vi "qc5psmCurrent1.vi"() -> ()   [LabVIEW 2020]
uses:
  <instrlib>/CAEN PSM/CAEN PSM.lvlib
panel:
  in  "Tab Control":enum32{"Page 1"}(tab)
  out "RAMPUP1TIME":dbl
  in  "Tab Control 2":enum32{"Page 1", "Page 2"}(tab)
  out "V monitor":dbl(graph)
  out "I monitor":dbl(graph)
  out "Actual voltage level (Vmon)":dbl
  out "Actual current level (Imon)":dbl
  in  "I_step":dbl=10.0
  in  "VISA resource name":refnum<visa-resource-name>
  in  "Voltage ramp up (0 V/s)":u16 max=999
  in  "Voltage Max (0.0 V)":u16 max=9999
  in  "Board Address":i8 max=31
  out "Vset_initial":dbl=100.0
  out "OVV 2":bool
  out "OVC 2":bool
  out "R calc":dbl
  in  "START AGAIN":bool
  out "Channel Status Array":T1(array[cluster])
  in  "Channel (0)":u8=1
  in  "Req (Mohm)":dbl=4.647
  out "I set status":dbl
  in  "stop":bool
  in  "I_initial":dbl=550.0
  in  "wait for user to next reading":bool
  in  "I _Max":dbl=730.0
  out "status":string
  out "ENTER TIME RAMP VAL":i32
  out "RDW":bool
  out "Actual I mon STOP":dbl
  out "In Range?":bool
  out "INNER  RAMP VAL":dbl
  out "CURRENT INCREASE/DECREASE  PER 1 VOLT":dbl
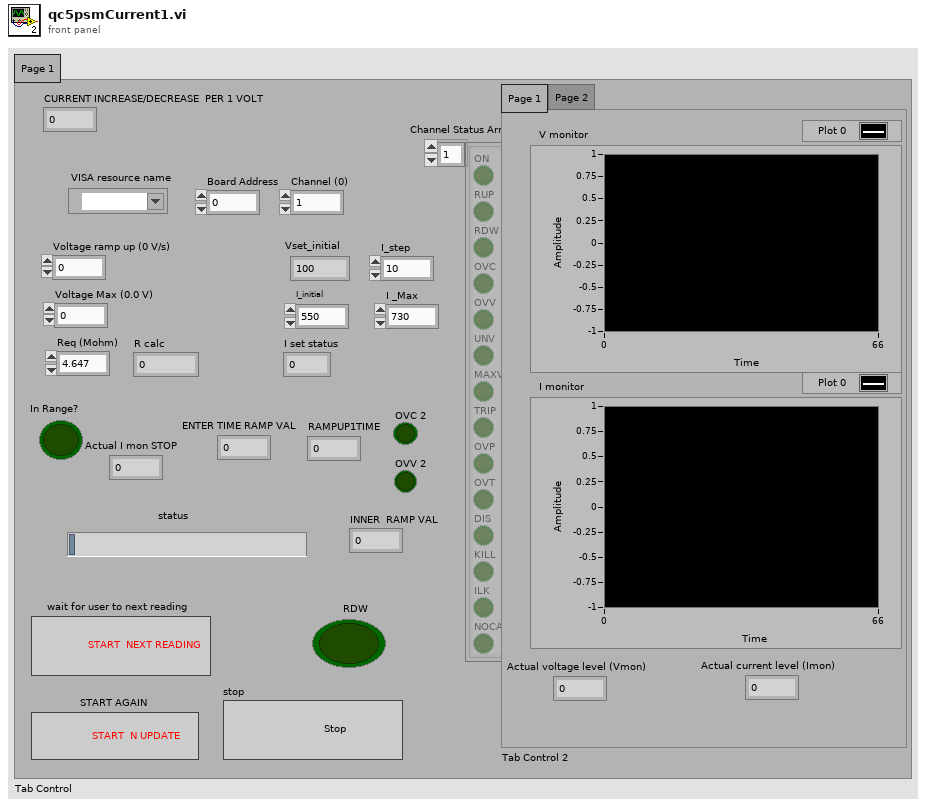
[diagram p1: front panel]
types:
  T1 = cluster{"ON":bool, "RUP":bool, "RDW":bool, "OVC":bool, "OVV":bool, "UNV":bool, "MAXV":bool, "TRIP":bool, "OVP":bool, "OVT":bool, "DIS":bool, "KILL":bool, "ILK":bool, "NOCAL":bool}[]
  T2 = cluster{"Baud Rate":u32, "Parity":enum16{"None", "Odd", "Even", "Mark", "Space"}, "Data Bits":u16, "Stop Bits":u16, "Flow Control":u16}
  T3 = typedef "CAEN PSM.lvlib/BoardHandle.ctl" = cluster{"VISA resource name":refnum<visa-resource-name>, "Board address":i8, "NChannels":u8}
  T4 = cluster{"ON":bool, "RUP":bool, "RDW":bool, "OVC":bool, "OVV":bool, "UNV":bool, "MAXV":bool, "TRIP":bool, "OVP":bool, "OVT":bool, "DIS":bool, "KILL":bool, "ILK":bool, "NOCAL":bool}
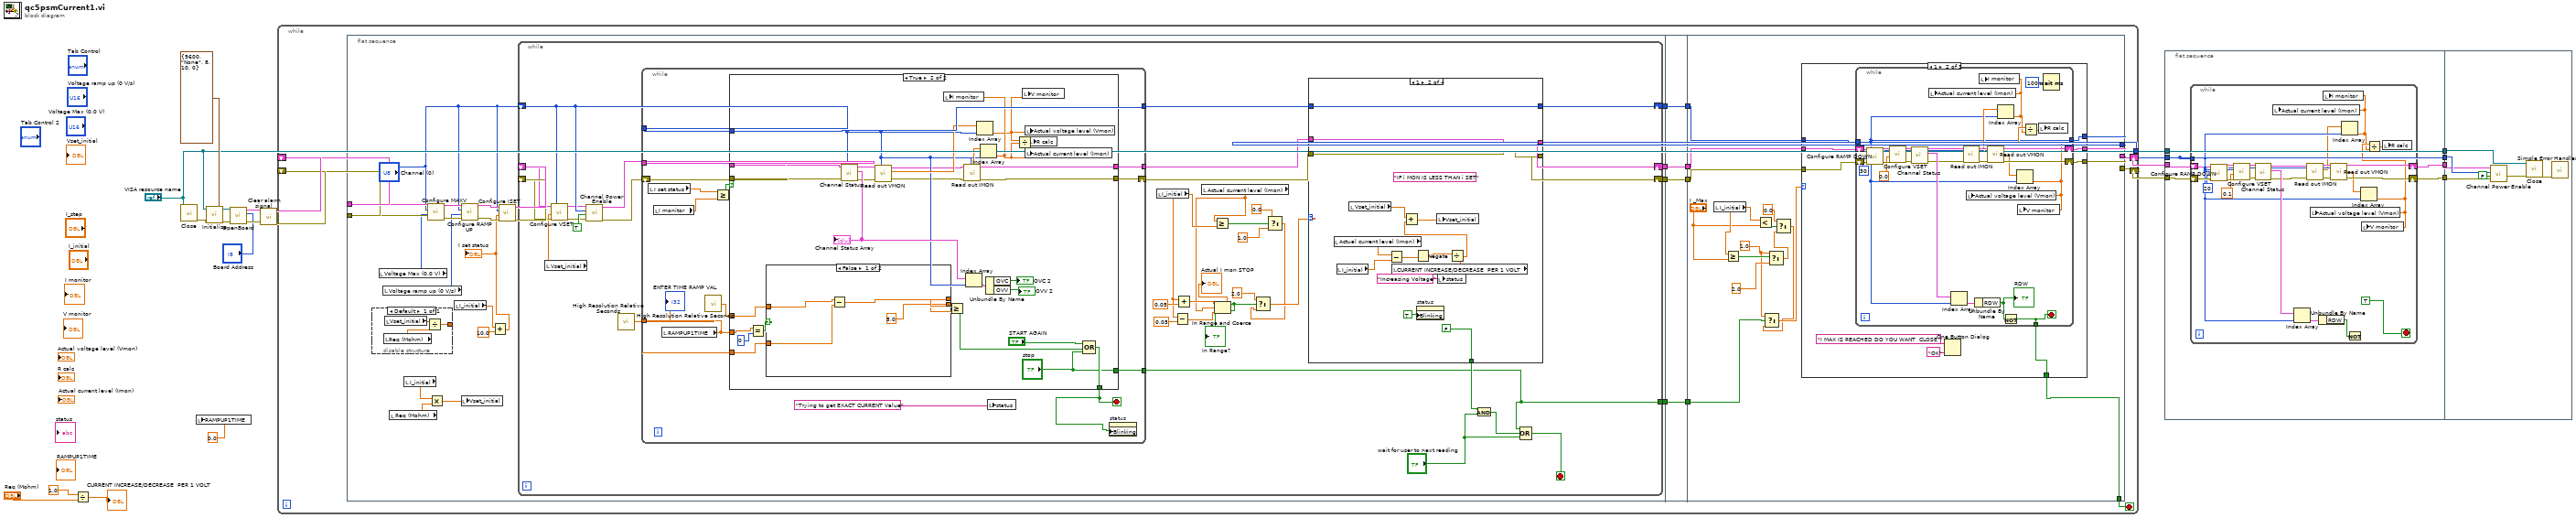
[diagram p0: block diagram]
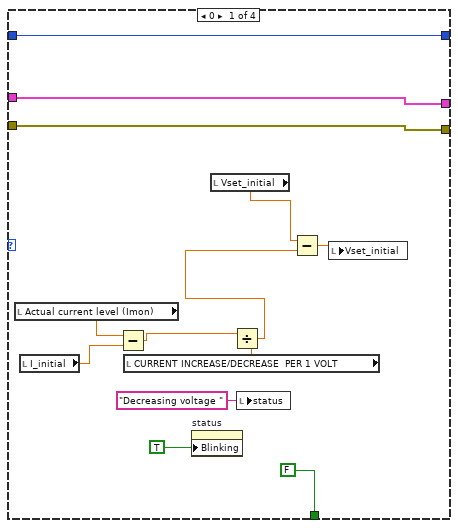
[diagram p2: hidden frame]
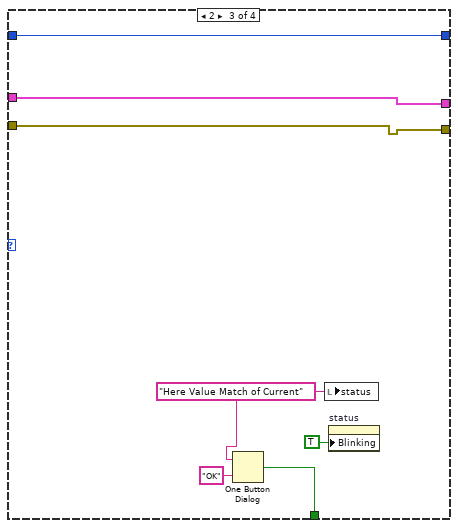
[diagram p3: hidden frame]
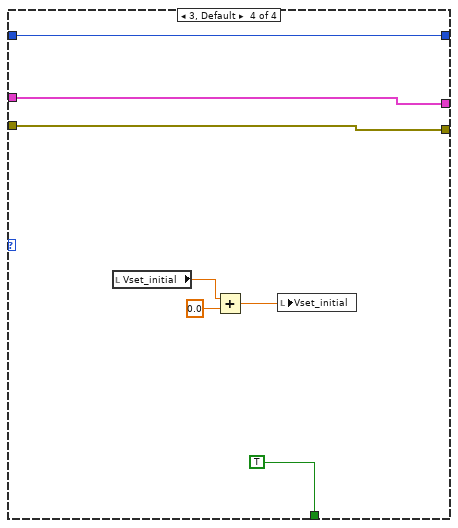
[diagram p4: hidden frame]
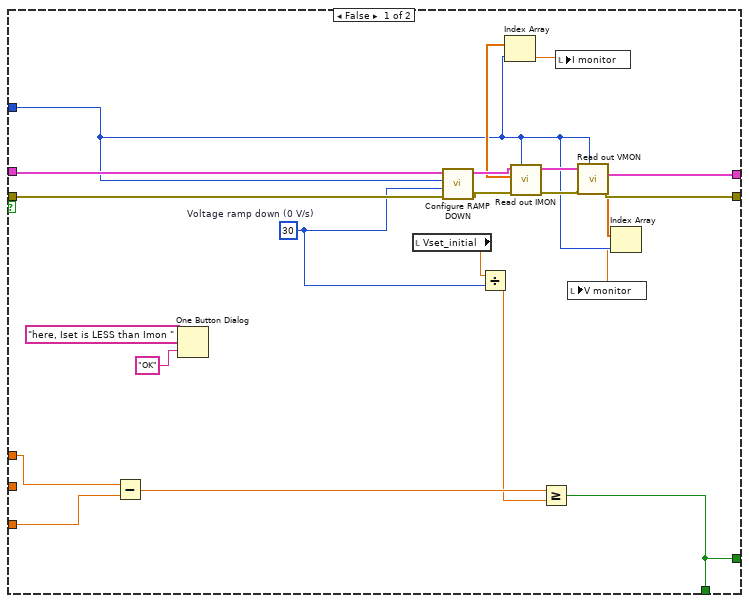
[diagram p5: hidden frame]
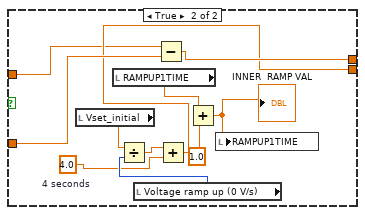
[diagram p6: hidden frame]
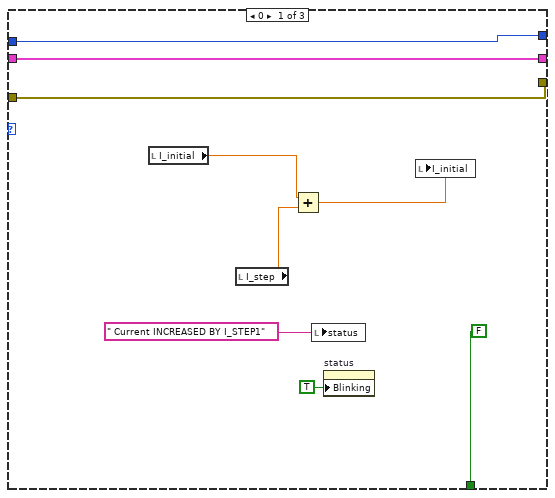
[diagram p7: hidden frame]
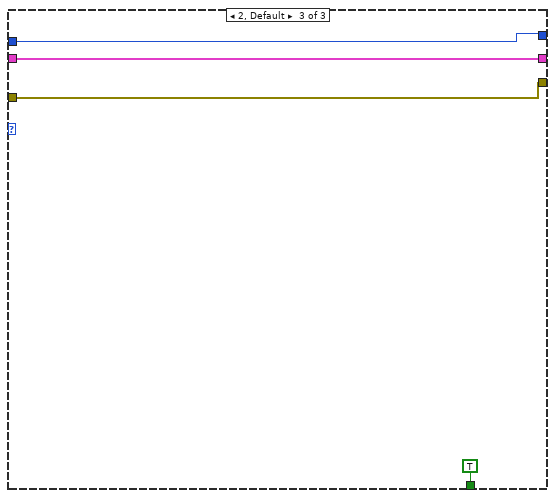
[diagram p8: hidden frame]
diagram:
  n1 = Divide(x=1.0, y="Req (Mohm)") -> (x/y=→"CURRENT INCREASE/DECREASE  PER 1 VOLT":dbl)
  n2 = call <instrlib>:"Close.vi"("VISA resource name"="VISA resource name") -> ("error out"=w12:errorcluster)  [unwired: 10 in]
  n3 = local write "RAMPUP1TIME"(0.0 ("RAMPUP1TIME")) -> ()
  n4 = call <instrlib>:"Initialize.vi"("Serial Configuration"=T2 {"Baud Rate"=9600, "Parity"=enum."None", "Data Bits"=8, "Stop Bits"=10, "Flow Control"=0}, "error in (no error)"=w12, "VISA resource name"="VISA resource name") -> ("error out"=w11:errorcluster, "VISA resource name out"=w20:refnum<visa-resource-name>)  [unwired: 7 in]
  n5 = call <instrlib>:"OpenBoard.vi"("error in (no error)"=w11, "Board Address"="Board Address", "VISA resource name"=w20) -> ("error out"=w18:errorcluster, "BoardHandle"=w19:T3)  [unwired: 7 in]
  n6 = call <instrlib>:"Clear alarm signal.vi"("error in (no error)"=w18, "BoardHandle"=w19) -> ("error out"=w13:errorcluster, "BoardHandle out"=w14:T3)  [unwired: 8 in]
  n7 = while {
    tunnel: [w35] -> w15
    shift-right: [w32] -> w10
    shift-left: w14 -> [w34]
    shift-right: [w30] -> w9
    shift-left: w13 -> [w33]
    stop <- w31 stop-if-true
    n8 = flat-sequence {
      tunnel: w34 -> [w55]
      tunnel: w33 -> [w54]
      tunnel: [w56] -> w25
      tunnel: [w43] -> w27
      tunnel: [w42] -> w29
      tunnel: [w36] -> w23
      tunnel: w29 -> [w219]
      tunnel: [w219] -> w28
      tunnel: w27 -> [w218]
      tunnel: [w218] -> w26
      tunnel: w25 -> [w217]
      tunnel: [w217] -> w24
      tunnel: w23 -> [w216]
      tunnel: [w216] -> w22
      tunnel: [w232] -> w30
      tunnel: [w231] -> w32
      tunnel: [w225] -> w35
      tunnel: [w224] -> w31
      tunnel: w28 -> [w229]
      tunnel: w26 -> [w228]
      tunnel: w24 -> [w230]
      tunnel: w22 -> [w223]
      frame #0 {
        n9 = disable-structure shown="Default" {
          disable-tunnel: [w59] -> _
          frame Enabled {
            n10 = local read "Req (Mohm)"() -> (w57:dbl)
            n11 = local read "Vset_initial"() -> (w58:dbl)
            n12 = Divide(x=w58, y=w57) -> (x/y=w59:dbl)
          }
        }
        n13 = local read "Voltage Max (0.0 V)"() -> (w51:u16)
        n14 = local read "Voltage ramp up (0 V/s)"() -> (w50:u16)
        n15 = local read "Req (Mohm)"() -> (w39:dbl)
        n16 = local read "I_initial"() -> (w38:dbl)
        n17 = call <instrlib>:"Configure MAXV.vi"("error in (no error)"=w54, "Voltage Max (0.0 V)"=w51, "Channel (0)"="Channel (0)", "BoardHandle"=w55) -> ("error out"=w52:errorcluster, "BoardHandle out"=w53:T3)  [unwired: 6 in]
        n18 = Multiply(x=w38, y=w39) -> (x*y=w40:dbl)
        n19 = local read "I_initial"() -> (w37:dbl)
        n20 = local write "Vset_initial"(w40) -> ()
        n21 = call <instrlib>:"Configure RAMP UP.vi"("error in (no error)"=w52, "Voltage ramp up (0 V/s)"=w50, "Channel (0)"="Channel (0)", "BoardHandle"=w53) -> ("error out"=w47:errorcluster, "BoardHandle out"=w49:T3)  [unwired: 6 in]
        n22 = Add(x=w37, y=10.0) -> (x+y=w41:dbl)
        "I set status" <- w41
        n23 = call <instrlib>:"Configure ISET.vi"("error in (no error)"=w47, "Current Limit (0.00 uA)"=w41, "Channel (0)"="Channel (0)", "BoardHandle"=w49) -> ("error out"=w46:errorcluster, "BoardHandle out"=w48:T3)  [unwired: 6 in]
        n24 = while {
          shift-right: [w73] -> w43
          shift-left: w48 -> [w91]
          shift-right: [w71] -> w42
          shift-left: w46 -> [w90]
          shift-right: [w75] -> w56
          shift-left: "Channel (0)" -> [w89]
          tunnel: [w77] -> w36
          stop <- w78 stop-if-true
          n25 = local read "Vset_initial"() -> (w83:dbl)
          n26 = call <instrlib>:"Configure VSET.vi"("error in (no error)"=w90, "Voltage Level (0.0 V)"=w83, "Channel (0)"=w89, "BoardHandle"=w91) -> ("error out"=w88:errorcluster, "BoardHandle out"=w87:T3)  [unwired: 6 in]
          n27 = call <instrlib>:"Channel Power Enable.vi"("error in (no error)"=w88, "Enable (OFF)"=TRUE, "Channel (0)"=w89, "BoardHandle"=w87) -> ("error out"=w93:errorcluster, "BoardHandle out"=w94:T3)  [unwired: 6 in]
          n28 = call <vilib>:"High Resolution Relative Seconds.vi"() -> ("relative seconds"=w86:dbl)
          n29 = while {
            shift-right: [w146] -> w72
            shift-left: w93 -> [w147]
            tunnel: [w145] -> w74
            tunnel: [w149] -> w76
            tunnel: w94 -> [w148]
            tunnel: w89 -> [w149]
            tunnel: w86 -> [w143]
            tunnel: [w139] -> w77
            stop <- w137 stop-if-true
            n30 = local read "I set status"() -> (w142:dbl)
            n31 = local read "I monitor"() -> (w140:dbl)
            n32 = local read "RAMPUP1TIME"() -> (w136:dbl)
            "ENTER TIME RAMP VAL" <- w136
            n33 = call <vilib>:"High Resolution Relative Seconds.vi"() -> ("relative seconds"=w141:dbl)
            n34 = Greater Or Equal?(x=w142, y=w140) -> (x >= y?=w144:bool)
            n35 = case shown="True" w144 {
              tunnel: w149 -> [w156 w194]
              tunnel: w148 -> [w171 w193]
              tunnel: w147 -> [w170 w192]
              tunnel: [w159 w191] -> w146
              tunnel: [w160 w190] -> w145
              tunnel: w143 -> [w169 w185]
              tunnel: [w150 w181] -> w137
              tunnel: w141 -> [w151 w176]
              tunnel: [w150 "stop"] -> w139
              tunnel: w136 -> [_ w172]
              frame False {
                w166 = u16 30  # Voltage ramp down (0 V/s)
                n36 = Subtract(x=w151, y=w169) -> (x-y=w168:dbl)
                n37 = One Button Dialog(message="here, Iset is LESS than Imon ", button name ("OK")="OK") -> ()  [unwired: 1 out]
                n38 = local read "Vset_initial"() -> (w167:dbl)
                n39 = call <instrlib>:"Configure RAMP DOWN.vi"("error in (no error)"=w170, "Voltage ramp down (0 V/s)"=w166, "Channel (0)"=w156, "BoardHandle"=w171) -> ("error out"=w163:errorcluster, "BoardHandle out"=w164:T3)  [unwired: 6 in]
                n40 = Divide(x=w167, y=w166) -> (x/y=w165:dbl)
                n41 = call <instrlib>:"Read out IMON.vi"("Channel"=w156, "error in (no error)"=w163, "BoardHandle"=w164) -> ("error out"=w161:errorcluster, "IMon values (uA)"=w158:dbl[], "BoardHandle out"=w162:T3)  [unwired: 5 in, 1 out]
                n42 = Index Array(array=w158, index=w156) -> (element=w153:dbl)
                n43 = Greater Or Equal?(x=w168, y=w165) -> (x >= y?=w150:bool)
                n44 = local write "I monitor"(w153) -> ()
                n45 = call <instrlib>:"Read out VMON.vi"("Channel"=w156, "error in (no error)"=w161, "BoardHandle"=w162) -> ("error out"=w159:errorcluster, "VMon values (V)"=w157:dbl[], "BoardHandle out"=w160:T3)  [unwired: 6 in]
                n46 = Index Array(array=w157, index=w156) -> (element=w152:dbl)
                n47 = local write "V monitor"(w152) -> ()
              }
              frame True {
                n48 = Equal?(x=w172, y=0) -> (x = y?=w174:bool)
                n49 = case shown="False" w174 {
                  tunnel: w185 -> [w203 w215]
                  tunnel: [w201 w214] -> w182
                  tunnel: [5.0 w209] -> w180
                  tunnel: w176 -> [w204 w208]
                  frame False {
                    n50 = Subtract(x=w204, y=w203) -> (x-y=w201:dbl)
                  }
                  frame True {
                    w210 = 4.0  # 4 seconds
                    n51 = local read "Vset_initial"() -> (w213:dbl)
                    n52 = local read "RAMPUP1TIME"() -> (w207:dbl)
                    n53 = local read "Voltage ramp up (0 V/s)"() -> (w212:u16)
                    n54 = Divide(x=w213, y=w212) -> (x/y=w211:dbl)
                    n55 = Subtract(x=w208, y=w215) -> (x-y=w214:dbl)
                    n56 = Add(x=w211, y=w210) -> (x+y=w209:dbl)
                    n57 = Add(x=w207, y=1.0) -> (x+y=w205:dbl)
                    "INNER  RAMP VAL" <- w205
                    n58 = local write "RAMPUP1TIME"(w205) -> ()
                  }
                }
                n59 = call <instrlib>:"Channel Status.vi"("Channel"=w194, "error in (no error)"=w192, "BoardHandle"=w193) -> ("error out"=w188:errorcluster, "Channel Status Array"=w199:T1, "BoardHandle out"=w189:T3)  [unwired: 5 in, 1 out]
                "Channel Status Array" <- w199
                n60 = call <instrlib>:"Read out VMON.vi"("Channel"=w194, "error in (no error)"=w188, "BoardHandle"=w189) -> ("error out"=w186:errorcluster, "VMon values (V)"=w200:dbl[], "BoardHandle out"=w187:T3)  [unwired: 6 in]
                n61 = Greater Or Equal?(x=w182, y=w180) -> (x >= y?=w184:bool)
                n62 = call <instrlib>:"Read out IMON.vi"("Channel"=w194, "error in (no error)"=w186, "BoardHandle"=w187) -> ("error out"=w191:errorcluster, "IMon values (uA)"=w195:dbl[], "BoardHandle out"=w190:T3)  [unwired: 5 in, 1 out]
                n63 = Index Array(array=w199, index=w194) -> (element=w198:T4)
                n64 = Index Array(array=w200, index=w194) -> (element=w177:dbl)
                n65 = Index Array(array=w195, index=w194) -> (element=w178:dbl)
                n66 = local write "I monitor"(w178) -> ()
                n67 = Unbundle By Name(w198) -> ("OVC"=→"OVC 2":bool, "OVV"=→"OVV 2":bool)
                n68 = Divide(x=w177, y=w178) -> (x/y=w179:dbl)
                n69 = local write "V monitor"(w177) -> ()
                n70 = local write "Actual voltage level (Vmon)"(w177) -> ()
                n71 = local write "Actual current level (Imon)"(w178) -> ()
                n72 = local write "R calc"(w179) -> ()
                n73 = Compound Arithmetic op=OR("START AGAIN", w184, "stop") -> (w181:bool)
              }
            }
            n74 = local write "status"("Trying to get EXACT CURRENT Value" ("status")) -> ()
            n75 = property on="status" class="Str"("Blinking"=w137) -> ()  [unwired: 2 in, 2 out]
          }
          n76 = local read "I_initial"() -> (w64:dbl)
          n77 = Subtract(x=w64, y=0.05) -> (x-y=w66:dbl)
          n78 = Add(x=w64, y=0.05) -> (x+y=w67:dbl)
          n79 = local read "Actual current level (Imon)"() -> (w63:dbl)
          n80 = Greater Or Equal?(x=w63, y=w64) -> (x >= y?=w85:bool)
          n81 = In Range and Coerce(upper limit=w67, x=w63, lower limit=w66) -> (coerced(x)=→"Actual I mon STOP":dbl, In Range?=w70:bool)
          "In Range?" <- w70
          n82 = Select(t=0.0, s=w85, f=1.0 ("t")) -> (s? t:f=w61:dbl)
          n83 = Select(t=2.0 ("f"), s=w70, f=w61) -> (s? t:f=w62:dbl)
          n84 = case shown="1" w62 {
            tunnel: [FALSE FALSE w124 TRUE] -> w81
            tunnel: w76 -> [w104 w118 w128 w131]
            tunnel: [w104 w118 w128 w131] -> w75
            tunnel: [w103 w117 w127 w130] -> w73
            tunnel: w74 -> [w103 w117 w127 w130]
            tunnel: [w102 w116 w126 w129] -> w71
            tunnel: w72 -> [w102 w116 w126 w129]
            frame 0 {
              n85 = local read "Actual current level (Imon)"() -> (w98:dbl)
              n86 = local read "I_initial"() -> (w99:dbl)
              n87 = Subtract(x=w98, y=w99) -> (x-y=w95:dbl)
              n88 = local read "CURRENT INCREASE/DECREASE  PER 1 VOLT"() -> (w97:dbl)
              n89 = property on="status" class="Str"("Blinking"=TRUE) -> ()  [unwired: 2 in, 2 out]
              n90 = local read "Vset_initial"() -> (w107:dbl)
              n91 = Divide(x=w95, y=w97) -> (x/y=w96:dbl)
              n92 = local write "status"("Decreasing voltage " ("status")) -> ()
              n93 = Subtract(x=w107, y=w96) -> (x-y=w106:dbl)
              n94 = local write "Vset_initial"(w106) -> ()
            }
            frame 1 {
              (unwired) "IF i MON IS LESS THAN i SET"
              n95 = local read "Actual current level (Imon)"() -> (w112:dbl)
              n96 = local read "I_initial"() -> (w113:dbl)
              n97 = local read "Vset_initial"() -> (w121:dbl)
              n98 = Subtract(x=w112, y=w113) -> (x-y=w111:dbl)
              n99 = local read "CURRENT INCREASE/DECREASE  PER 1 VOLT"() -> (w109:dbl)
              n100 = Negate(x=w111) -> (-x=w110:dbl)
              n101 = property on="status" class="Str"("Blinking"=TRUE) -> ()  [unwired: 2 in, 2 out]
              n102 = local write "status"("Increasing Voltage" ("status")) -> ()
              n103 = Divide(x=w110, y=w109) -> (x/y=w108:dbl)
              n104 = Add(x=w121, y=w108) -> (x+y=w120:dbl)
              n105 = local write "Vset_initial"(w120) -> ()
            }
            frame 2 {
              w123 = "Here Value Match of Current" ("status")
              n106 = One Button Dialog(message=w123, button name ("OK")="OK") -> (true=w124:bool)
              n107 = local write "status"(w123) -> ()
              n108 = property on="status" class="Str"("Blinking"=TRUE) -> ()  [unwired: 2 in, 2 out]
            }
            frame 3, Default {
              n109 = local read "Vset_initial"() -> (w135:dbl)
              n110 = Add(x=w135, y=0.0) -> (x+y=w133:dbl)
              n111 = local write "Vset_initial"(w133) -> ()
            }
          }
          n112 = Compound Arithmetic op=AND(w81, "wait for user to next reading") -> (w80:bool)
          n113 = Compound Arithmetic op=OR(w77, w80, "wait for user to next reading") -> (w78:bool)
        }
      }
      frame #1 {
      }
      frame #2 {
        w222 = 1.0 ("t")
        n114 = local read "I_initial"() -> (w227:dbl)
        n115 = Greater Or Equal?(x=w227, y="I _Max") -> (x >= y?=w235:bool)
        n116 = Less?(x=w227, y="I _Max") -> (x < y?=w237:bool)
        n117 = Select(t=w222, s=w235, f=2.0) -> (s? t:f=w234:dbl)
        n118 = Select(t=0.0, s=w237, f=w234) -> (s? t:f=w220:dbl)
        n119 = Select(t=w222, s=w223, f=w220) -> (s? t:f=w221:dbl)
        n120 = case shown="1" w221 {
          tunnel: [FALSE w250 TRUE] -> w224
          tunnel: w230 -> [w243 w255 w281]
          tunnel: w228 -> [w245 w254 w283]
          tunnel: w229 -> [w244 w253 w282]
          tunnel: [w244 w251 w282] -> w232
          tunnel: [w245 w252 w283] -> w231
          tunnel: [w243 w247 w281] -> w225
          frame 0 {
            n121 = local read "I_initial"() -> (w241:dbl)
            n122 = local read "I_step"() -> (w242:dbl)
            n123 = Add(x=w241, y=w242) -> (x+y=w240:dbl)
            n124 = local write "status"(" Current INCREASED BY I_STEP1" ("status")) -> ()
            n125 = property on="status" class="Str"("Blinking"=TRUE) -> ()  [unwired: 2 in, 2 out]
            n126 = local write "I_initial"(w240) -> ()
          }
          frame 1 {
            n127 = while {
              tunnel: w255 -> [w257]
              shift-right: [w277] -> w252
              shift-left: w254 -> [w279]
              shift-right: [w276] -> w251
              shift-left: w253 -> [w278]
              tunnel: [w257] -> w247
              tunnel: [w256] -> w250
              stop <- w256 stop-if-true
              n128 = call <instrlib>:"Configure RAMP DOWN.vi"("error in (no error)"=w278, "Voltage ramp down (0 V/s)"=u16 30, "Channel (0)"=w257, "BoardHandle"=w279) -> ("error out"=w272:errorcluster, "BoardHandle out"=w273:T3)  [unwired: 6 in]
              n129 = call <instrlib>:"Configure VSET.vi"("error in (no error)"=w272, "Voltage Level (0.0 V)"=0.0, "Channel (0)"=w257, "BoardHandle"=w273) -> ("error out"=w269:errorcluster, "BoardHandle out"=w270:T3)  [unwired: 6 in]
              n130 = call <instrlib>:"Channel Status.vi"("Channel"=w257, "error in (no error)"=w269, "BoardHandle"=w270) -> ("error out"=w264:errorcluster, "Channel Status Array"=w268:T1, "BoardHandle out"=w263:T3)  [unwired: 5 in, 1 out]
              n131 = Index Array(array=w268, index=w257) -> (element=w267:T4)
              n132 = call <instrlib>:"Read out IMON.vi"("Channel"=w257, "BoardHandle"=w263) -> ("IMon values (uA)"=w261:dbl[], "BoardHandle out"=w262:T3)  [unwired: 6 in, 2 out]
              n133 = Unbundle By Name(w267) -> ("RDW"=w266:bool)
              "RDW" <- w266
              n134 = call <instrlib>:"Read out VMON.vi"("Channel"=w257, "error in (no error)"=w264, "BoardHandle"=w262) -> ("error out"=w276:errorcluster, "VMon values (V)"=w274:dbl[], "BoardHandle out"=w277:T3)  [unwired: 6 in]
              n135 = Index Array(array=w261, index=w257) -> (element=w258:dbl)
              n136 = local write "Actual current level (Imon)"(w258) -> ()
              n137 = local write "I monitor"(w258) -> ()
              n138 = Not(x=w266) -> (.not. x?=w256:bool)
              n139 = Index Array(array=w274, index=w257) -> (element=w259:dbl)
              n140 = local write "Actual voltage level (Vmon)"(w259) -> ()
              n141 = local write "V monitor"(w259) -> ()
              n142 = Divide(x=w259, y=w258) -> (x/y=w260:dbl)
              n143 = local write "R calc"(w260) -> ()
              n144 = Wait (ms)(milliseconds to wait=u32 100) -> ()  [unwired: 1 out]
            }
            n145 = One Button Dialog(message="I MAX IS REACHED DO YOU WANT  CLOSE ", button name ("OK")="OK") -> ()  [unwired: 1 out]
          }
          frame 2, Default {
          }
        }
      }
    }
  }
  n146 = flat-sequence {
    tunnel: w9 -> [w287]
    tunnel: w10 -> [w288]
    tunnel: w15 -> [w284]
    tunnel: "VISA resource name" -> [w289]
    tunnel: [w289] -> w8
    tunnel: [w284] -> w7
    tunnel: [w286] -> w6
    tunnel: [w285] -> w5
    tunnel: w8 -> [w317]
    tunnel: w7 -> [w315]
    tunnel: w6 -> [w314]
    tunnel: w5 -> [w313]
    frame #0 {
      n147 = while {
        tunnel: w284 -> [w300]
        shift-right: [w310] -> w286
        shift-left: w288 -> [w312]
        shift-right: [w309] -> w285
        shift-left: w287 -> [w311]
        stop <- TRUE stop-if-true
        n148 = call <instrlib>:"Configure RAMP DOWN.vi"("error in (no error)"=w311, "Voltage ramp down (0 V/s)"=u16 20, "Channel (0)"=w300, "BoardHandle"=w312) -> ("error out"=w305:errorcluster, "BoardHandle out"=w306:T3)  [unwired: 6 in]
        n149 = call <instrlib>:"Configure VSET.vi"("error in (no error)"=w305, "Voltage Level (0.0 V)"=0.1, "Channel (0)"=w300, "BoardHandle"=w306) -> ("error out"=w302:errorcluster, "BoardHandle out"=w303:T3)  [unwired: 6 in]
        n150 = call <instrlib>:"Channel Status.vi"("Channel"=w300, "error in (no error)"=w302, "BoardHandle"=w303) -> ("error out"=w297:errorcluster, "Channel Status Array"=w301:T1, "BoardHandle out"=w296:T3)  [unwired: 5 in, 1 out]
        n151 = Index Array(array=w301, index=w300) -> (element=w299:T4)
        n152 = call <instrlib>:"Read out IMON.vi"("Channel"=w300, "BoardHandle"=w296) -> ("IMon values (uA)"=w294:dbl[], "BoardHandle out"=w295:T3)  [unwired: 6 in, 2 out]
        n153 = Unbundle By Name(w299) -> ("RDW"=w298:bool)
        n154 = call <instrlib>:"Read out VMON.vi"("Channel"=w300, "error in (no error)"=w297, "BoardHandle"=w295) -> ("error out"=w309:errorcluster, "VMon values (V)"=w307:dbl[], "BoardHandle out"=w310:T3)  [unwired: 6 in]
        n155 = Index Array(array=w294, index=w300) -> (element=w291:dbl)
        n156 = local write "Actual current level (Imon)"(w291) -> ()
        n157 = local write "I monitor"(w291) -> ()
        n158 = Not(x=w298) -> ()  [unwired: 1 out]
        n159 = Index Array(array=w307, index=w300) -> (element=w292:dbl)
        n160 = local write "Actual voltage level (Vmon)"(w292) -> ()
        n161 = local write "V monitor"(w292) -> ()
        n162 = Divide(x=w292, y=w291) -> (x/y=w293:dbl)
        n163 = local write "R calc"(w293) -> ()
      }
    }
    frame #1 {
      n164 = call <instrlib>:"Channel Power Enable.vi"("error in (no error)"=w313, "Enable (OFF)"=FALSE, "Channel (0)"=w315, "BoardHandle"=w314) -> ("error out"=w319:errorcluster)  [unwired: 6 in, 1 out]
      n165 = call <instrlib>:"Close.vi"("error in (no error)"=w319, "VISA resource name"=w317) -> ("error out"=w318:errorcluster)  [unwired: 9 in]
      n166 = call <vilib>:"Simple Error Handler.vi"("error in (no error)"=w318) -> ()  [unwired: 4 in, 5 out]
    }
  }
